vi "str appendchar.vi"(8 "error in (no error)":errorcluster, 9 "C":i8, 10 "N":i32, 11 "para0":dbl) -> (0 "error out":errorcluster, 3 "para0 out":dbl)   [LabVIEW 2020, in "sqlite3.lvlib"]
uses:
  sqlite3.lvlib
  errstr.vi
  bin/sqlite3_64.dll
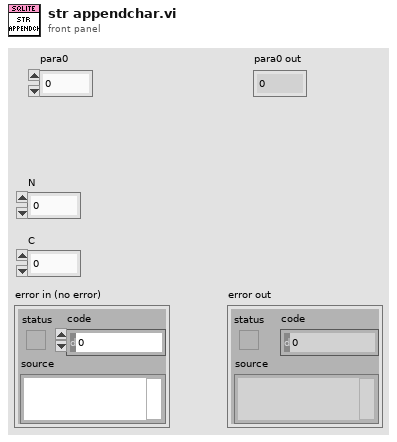
[diagram p1: front panel]
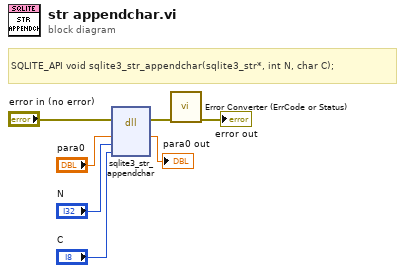
[diagram p0: block diagram]
diagram:
  # "SQLITE_API void sqlite3_str_appendchar(sqlite3_str*, int N, char C);"
  n1 = dll-call lib="C:/Users/Fred.Guo/Desktop/Database-configuration/externals/sqlite3/Source/bin/sqlite3_*.*" fn="sqlite3_str_appendchar"(error in="error in (no error)", "para0"="para0", "N"="N", "C"="C") -> (error out=w2:errorcluster, "para0"=→"para0 out":dbl)  [unwired: 5 in, 1 out]
  n2 = call "Error Converter (ErrCode or Status).vi"("error in (no error)"=w2) -> ("error out"=→"error out":errorcluster)  [unwired: 10 in]
